vi "CreateStopEvent.vi"(8 "error in (no error)":errorcluster, 11 "TCP_Client in":refnum<class "TCP_Client.lvclass">) -> (0 "error out":errorcluster, 2 "Event Registration Refnum":refnum<event-registration>, 3 "TCP_Client out":refnum<class "TCP_Client.lvclass">)   [LabVIEW 2023, in "TCP_Client.lvlib" / "TCP_Client.lvclass"]
uses:
  TCP_Client.lvclass
  TCP_Client.lvclass/TCP_Client.ctl
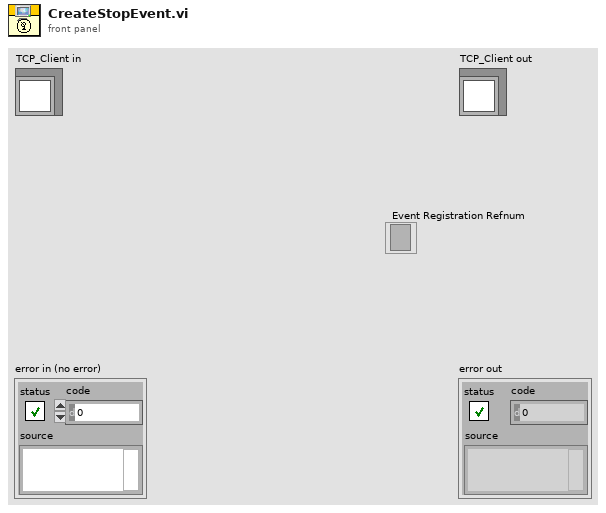
[diagram p1: front panel]
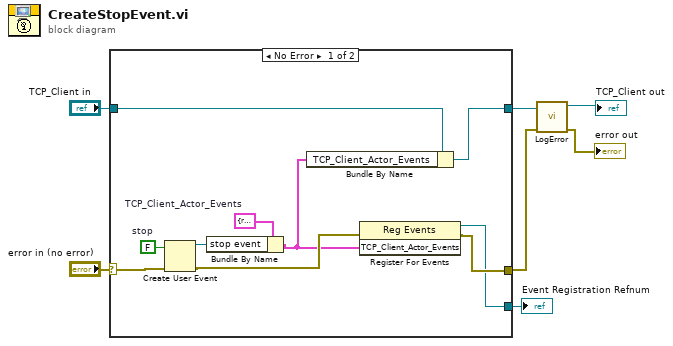
[diagram p0: block diagram]
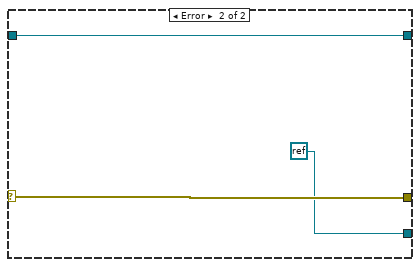
[diagram p2: hidden frame]
diagram:
  n1 = case shown="No Error" "error in (no error)" {
    selector: "error in (no error)" -> [w17 w20]
    tunnel: [w9 w20] -> w2
    tunnel: [w10 w19] -> w4
    tunnel: "TCP_Client in" -> [w12 w19]
    tunnel: [w8 refnum<k0> refnum] -> w5
    frame No Error {
      w15 = cluster{"stop event":refnum<user-event>} {"stop event"=refnum}  # TCP_Client_Actor_Events
      w16 = FALSE  # stop
      n2 = Create User Event(user event datatype=w16, error in=w17) -> (user event=w14:refnum<user-event>, error out=w13:errorcluster)
      n3 = Bundle By Name(cluster=w15, "stop event"=w14) -> (w11:cluster{"stop event":refnum<user-event>})
      n4 = Bundle By Name(cluster=w12, "TCP_Client_Actor_Events"=w11) -> (w10:refnum<class "TCP_Client.lvclass">)
      n5 = register-events(error in=w13, w11) -> (reference out=w8:refnum<event-registration>, error out=w9:errorcluster)  [unwired: 1 in]
    }
    frame Error {
    }
  }
  "Event Registration Refnum" <- w5
  n6 = call "LogError.vi"("error in (no error)"=w2, "TCP_Client in"=w4) -> ("error out"=→"error out":errorcluster, "TCP_Client out"=→"TCP_Client out":refnum<class "TCP_Client.lvclass">)  [unwired: 8 in]
